vi "Begin[Conflict].vi"() -> (0 "Joystick 1 Error":errorcluster)   [LabVIEW 2013]
doc: "Called before other user functions, this VI is expected to open initial I/O refnums, load in file data, and do all program initialization. Notice that the <B>error out</B> terminal is simply used for data flow. Wiring it to other structures or subVIs ensures that this VI runs first."
uses:
  <vilib>/Rock Robotics/SystemInterfaces/DIO/FPGA_DIOPWMChannel.ctl
  <vilib>/Rock Robotics/WPI/SafetyOutput/WPI_SafetyOutputConfigMenu.ctl
  <vilib>/Rock Robotics/WPI/DriverStation/WPI_DriverStationRobotMode2.ctl
  <vilib>/Rock Robotics/SystemInterfaces/Typedef/FPGA_TypedefAnalogModuleForGyro.ctl
  <vilib>/Rock Robotics/SystemInterfaces/AI/FPGA_AIGyroChannel.ctl
  <vilib>/Rock Robotics/WPI/Solenoid/WPI_SolenoidChannel.ctl
  <vilib>/Rock Robotics/SystemInterfaces/DIO/FPGA_DIOChannel.ctl
  <vilib>/Rock Robotics/SystemInterfaces/DIO/FPGA_DIORelayChannel.ctl
  <vilib>/Rock Robotics/WPI/Relay/WPI_RelayDirection.ctl
  <vilib>/Rock Robotics/SystemInterfaces/Typedef/FPGA_TypedefSolenoidModule.ctl
  <vilib>/Rock Robotics/WPI/Joystick/WPI_JoystickDeviceEnum.ctl
  <vilib>/Rock Robotics/WPI/RobotDrive/WPI_RobotDriveOpen2MotorWithTalon.vi
  Robot Global Data.vi
  <vilib>/Rock Robotics/WPI/Solenoid/WPI_SolenoidOpenDouble.vi
panel:
  out "TestSolenoid56":errorcluster
  out "Test Gripper Error":errorcluster
  out "Right Solenoid Open Error":errorcluster
  out "Left Solenoid Open Error":errorcluster
  out "Extsionsion Solenoids Error":errorcluster
  out "Catapult Solenoids Error":errorcluster
  out "Gripper Solenoid Open Error":errorcluster
  out "Joystick 3 Error":errorcluster
  out "Gyro Open Error":errorcluster
  out "Joystick 1 Error 2":errorcluster
  out "Compressor Open Error":errorcluster
  out "Joystick 2 Error":errorcluster
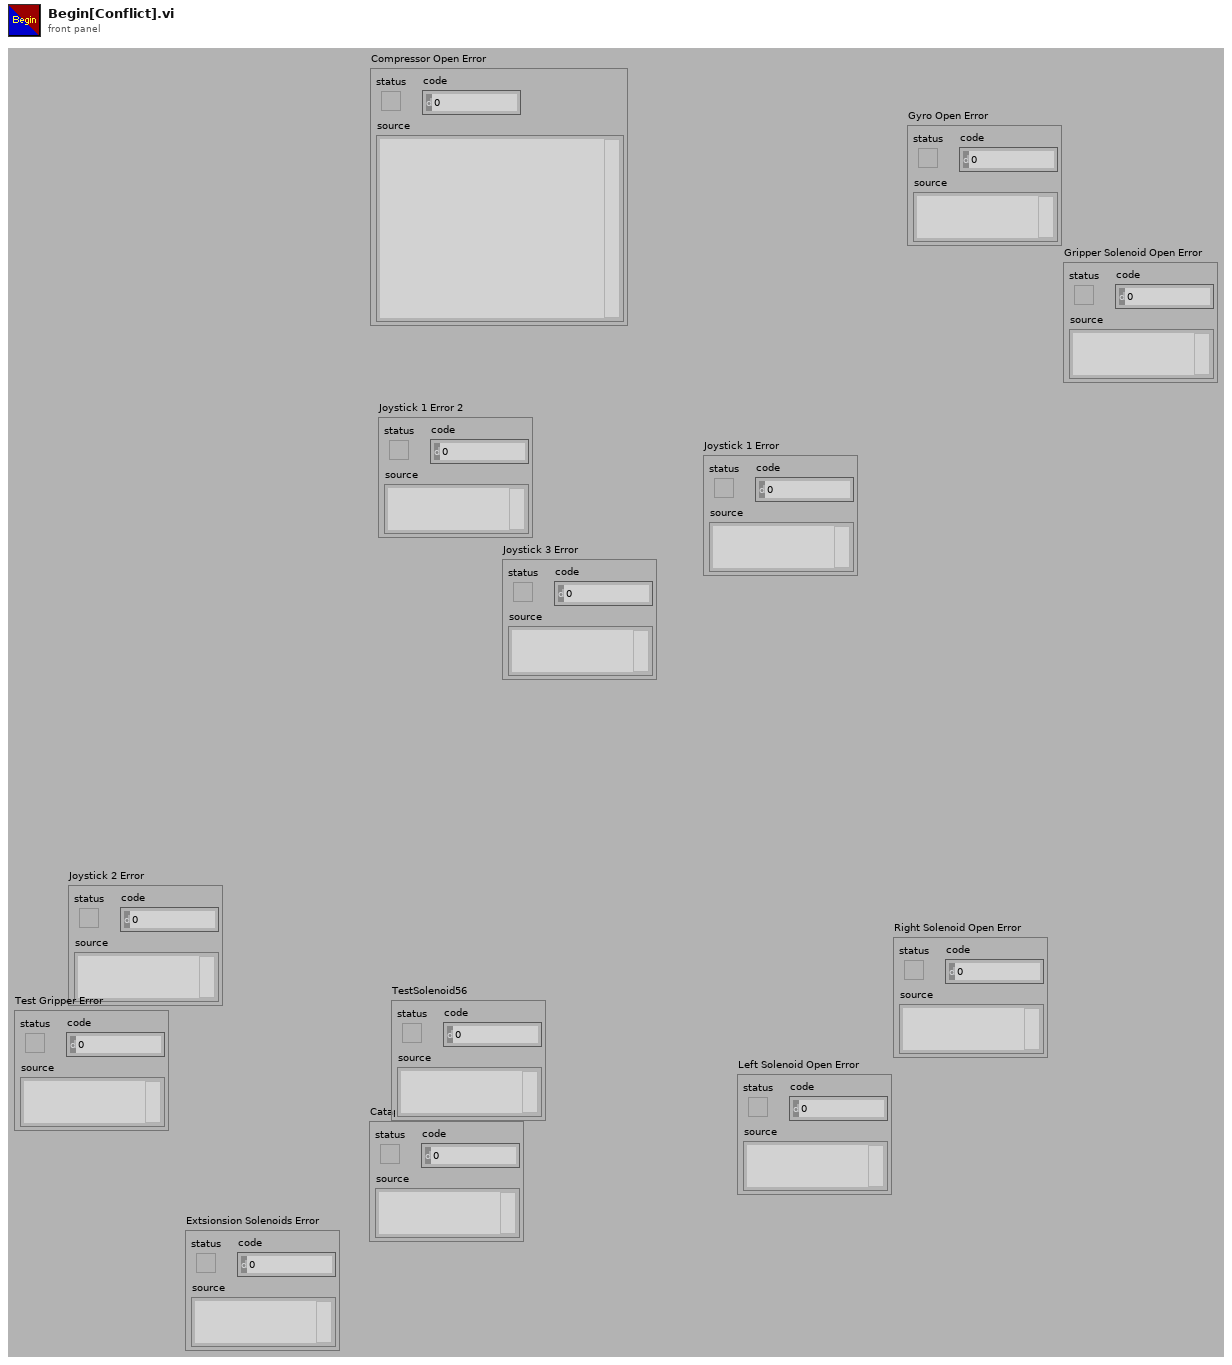
[diagram p1: front panel]
types:
  T1 = typedef "WPI_SolenoidChannel.ctl" = enum8{"Solenoid 1", "Solenoid 2", "Solenoid 3", "Solenoid 4", "Solenoid 5", "Solenoid 6", "Solenoid 7", "Solenoid 8", "Invalid"}
  T2 = typedef "FPGA_TypedefSolenoidModule.ctl" = enum16{"Solenoid Module 1", "Solenoid Module 2"}
  T3 = typedef "WPI_RelayDirection.ctl" = enum16{"Both directions", "Forward only", "Reverse only"}
  T4 = typedef "FPGA_DIORelayChannel.ctl" = enum8{"Relay 1", "Relay 2", "Relay 3", "Relay 4", "Relay 5", "Relay 6", "Relay 7", "Relay 8", "Invalid"}
  T5 = typedef "FPGA_DIOChannel.ctl" = enum8{"DIO 1", "DIO 2", "DIO 3", "DIO 4", "DIO 5", "DIO 6", "DIO 7", "DIO 8", "DIO 9", "DIO 10", "DIO 11", "DIO 12", "DIO 13", "DIO 14", "Invalid"}
  T6 = typedef "FPGA_AIGyroChannel.ctl" = enum8{"AI 1", "AI 2", "Invalid"}
  T7 = typedef "FPGA_TypedefAnalogModuleForGyro.ctl" = enum16{"Analog Module 1"}
  T8 = typedef "WPI_DriverStationRobotMode2.ctl" = enum16{"Autonomous Disabled", "Autonomous Enabled", "Teleop Disabled", "Teleop Enabled", "Timeout", "Finish", "Test Disabled", "Test Enabled"}
  T9 = typedef "WPI_SafetyOutputConfigMenu.ctl" = enum16{"Enable", "Disable"}
  T10 = typedef "FPGA_DIOPWMChannel.ctl" = enum8{"PWM 1", "PWM 2", "PWM 3", "PWM 4", "PWM 5", "PWM 6", "PWM 7", "PWM 8", "PWM 9", "PWM 10", "Invalid"}
  T11 = typedef "WPI_RobotDriveDevRef.ctl" = cluster{"DevStatus":errorcluster, "Motors[]":T12[], "Square Inputs":bool, "Max Output":dbl, "Isochronous":bool}
  T12 = typedef "WPI_MotorControlDeviceRef.ctl" = cluster{"DeviceStatus":errorcluster, "Type":enum16{"PWM", "CAN"}, "PWM":cluster{"Digital Module":T13, "PWM Channel":T10, "DeadBand":T14}, "CAN":cluster{"Device Number":u8, "Control Mode":T15, "Semaphore":T16, "Max Vout":dbl}, "Invert":bool, "TransformRef":T17, "InvTransformRef":T17}
  T13 = typedef "FPGA_TypedefDigitalModule.ctl" = enum16{"Digital Module 1", "Digital Module 2"}
  T14 = typedef "WPI_PWMDeadband.ctl" = cluster{"Name":string, "maxPositivePwm":i32, "minPositivePwm":i32, "centerPwm":i32, "maxNegativePwm":i32, "minNegativePwm":i32, "angularRange":u16}
  T15 = typedef "WPI_CANJaguar_ControlMode.ctl" = enum8{"Percent VBus", "Current", "Speed", "Position", "Voltage"}
  T16 = typedef "Semaphore RefNum" = refnum<k1>
  T17 = typedef "WPI_PWMTransform_ConPane.ctl" = refnum<vi>
  T18 = typedef "WPI_SolenoidDevRef.ctl" = cluster{"DevStatus":errorcluster, "Solenoid Module":T2, "Forward Solenoid Channel":T1, "Reverse Solenoid Channel":T1}
  T19 = typedef "WPI_JoystickDeviceEnum.ctl" = enum16{"USB 1", "USB 2", "USB 3", "USB 4", "Kinect 1", "Kinect 2"}
  T20 = typedef "WPI_JoystickDevRef.ctl" = cluster{"Device":T19}
  T21 = typedef "WPI_RelayDevRef.ctl" = cluster{"DevStatus":errorcluster, "Relay Channel":T4, "Digital Module":T13, "Relay Direction":T3}
  T22 = typedef "WPI_GyroDevRef.ctl" = cluster{"DevStatus":errorcluster, "Analog Module":T23, "Analog Channel":T24, "Offset":dbl, "Gain (VoltsPerDegree/Second)":dbl}
  T23 = typedef "FPGA_TypedefAnalogModule.ctl" = enum16{"Analog Module 1", "Analog Module 2"}
  T24 = typedef "FPGA_AIChannel.ctl" = enum8{"AI 1", "AI 2", "AI 3", "AI 4", "AI 5", "AI 6", "AI 7", "AI 8", "Invalid"}
  T25 = typedef "WPI_DigitalInputDevRef.ctl" = cluster{"DevStatus":errorcluster, "DIO Channel":T5, "Digital Module":T13}
  T26 = typedef "WPI_CompressorDevRef.ctl" = cluster{"DevStatus":errorcluster, "DigitalInputDevRef":T25, "RelayDevRef":T21}
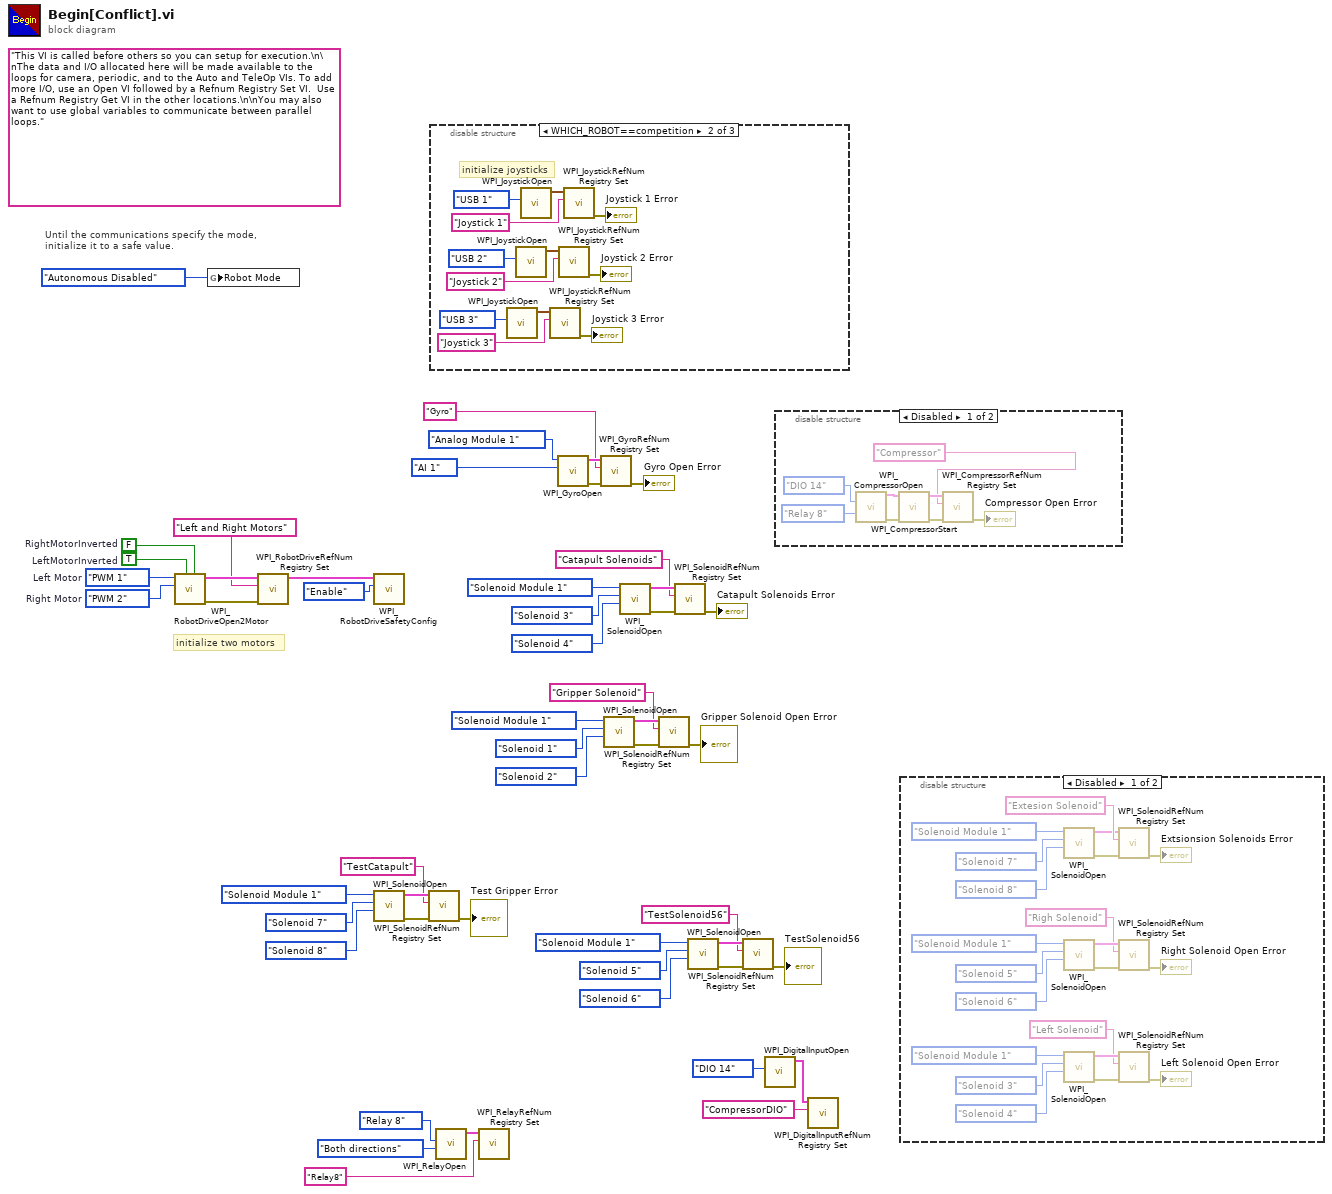
[diagram p0: block diagram]
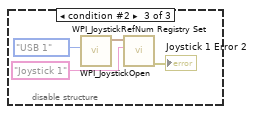
[diagram p5: hidden frame]
diagram:
  (unwired) "This VI is called before others so you can setup for execution.\n\nThe data and I/O allocated here will be made available to the loops for camera, periodic, and to the Auto and TeleOp VIs. To add more I/O, use an Open VI followed by a Refnum Registry Set VI.  Use a Refnum Registry Get VI in the other locations.\n\nYou may also want to use global variables to communicate between parallel loops."
  w45 = FPGA_DIOPWMChannel."PWM 2"  # Right Motor
  w46 = FPGA_DIOPWMChannel."PWM 1"  # Left Motor
  w50 = TRUE  # LeftMotorInverted
  w51 = FALSE  # RightMotorInverted
  # "Until the communications specify the mode,\ninitialize it to a safe value."
  # "initialize two motors"
  n1 = call-poly <vilib>:"WPI_RobotDriveOpen2Motor.vi"("Right Motor Inverted"=w51, "Left Motor Inverted"=w50, "Right Motor"=w45, "Left Motor"=w46) -> ("error out"=w47:errorcluster, "RobotDriveDevRef"=w49:T11)  [unwired: 1 in, 5 out]
  n2 = global write "Robot Global Data.vi" "Robot Mode"(WPI_DriverStationRobotMode2."Autonomous Disabled" ("Robot Mode")) -> ()
  n3 = call <vilib>:"WPI_RobotDriveRefNum Registry Set.vi"("error in (no error)"=w47, "refnum name"="Left and Right Motors", "RobotDriveDevRef"=w49) -> ("RobotDriveDevRef"=w44:T11)  [unwired: 8 out]
  n4 = call <vilib>:"WPI_RobotDriveSafetyConfig.vi"("mode"=WPI_SafetyOutputConfigMenu."Enable", "RobotDriveDevRef"=w44) -> ()  [unwired: 8 in, 2 out]
  n5 = call-poly <vilib>:"WPI_SolenoidOpen.vi"("Reverse Solenoid Channel"=WPI_SolenoidChannel."Solenoid 8", "Forward Solenoid Channel"=WPI_SolenoidChannel."Solenoid 7", "Solenoid Module (Module 1)"=FPGA_TypedefSolenoidModule."Solenoid Module 1") -> ("error out"=w10:errorcluster, "SolenoidDevRef"=w11:T18)  [unwired: 7 in]
  n6 = call <vilib>:"WPI_SolenoidRefNum Registry Set.vi"("error in (no error)"=w10, "refnum name"="TestCatapult", "SolenoidDevRef"=w11) -> ("error out"=→"Test Gripper Error":errorcluster)  [unwired: 7 in, 1 out]
  n7 = disable-structure shown="WHICH_ROBOT==competition" {
    frame condition #0 {
    }
    frame condition #1 (active) {
      # "initialize joysticks"
      n8 = call <vilib>:"WPI_JoystickOpen.vi"("JoystickDevice"=WPI_JoystickDeviceEnum."USB 3") -> ("JoystickDevRef"=w53:T20)  [unwired: 10 in]
      n9 = call <vilib>:"WPI_JoystickOpen.vi"("JoystickDevice"=WPI_JoystickDeviceEnum."USB 2") -> ("JoystickDevRef"=w61:T20)  [unwired: 10 in]
      n10 = call <vilib>:"WPI_JoystickOpen.vi"("JoystickDevice"=WPI_JoystickDeviceEnum."USB 1") -> ("JoystickDevRef"=w57:T20)  [unwired: 10 in]
      n11 = call <vilib>:"WPI_JoystickRefNum Registry Set.vi"("refnum name"="Joystick 3", "JoystickDevRef"=w53) -> ("error out"=→"Joystick 3 Error":errorcluster)  [unwired: 8 in, 1 out]
      n12 = call <vilib>:"WPI_JoystickRefNum Registry Set.vi"("refnum name"="Joystick 2", "JoystickDevRef"=w61) -> ("error out"=→"Joystick 2 Error":errorcluster)  [unwired: 8 in, 1 out]
      n13 = call <vilib>:"WPI_JoystickRefNum Registry Set.vi"("refnum name"="Joystick 1", "JoystickDevRef"=w57) -> ("error out"=→"Joystick 1 Error":errorcluster)  [unwired: 8 in, 1 out]
    }
    frame condition #2 {
      n14 = call <vilib>:"WPI_JoystickOpen.vi"("JoystickDevice"=WPI_JoystickDeviceEnum."USB 1") -> ("JoystickDevRef"=w65:T20)  [unwired: 10 in]
      n15 = call <vilib>:"WPI_JoystickRefNum Registry Set.vi"("refnum name"="Joystick 1", "JoystickDevRef"=w65) -> ("error out"=→"Joystick 1 Error 2":errorcluster)  [unwired: 8 in, 1 out]
    }
  }
  n16 = call <vilib>:"WPI_RelayOpen.vi"("Relay Direction"=WPI_RelayDirection."Both directions", "Relay Channel"=FPGA_DIORelayChannel."Relay 8") -> ("RelayDevRef"=w16:T21)  [unwired: 8 in, 1 out]
  n17 = call <vilib>:"WPI_RelayRefNum Registry Set.vi"("refnum name"="Relay8", "RelayDevRef"=w16) -> ()  [unwired: 8 in, 2 out]
  n18 = call <vilib>:"WPI_GyroOpen.vi"("Analog Channel"=FPGA_AIGyroChannel."AI 1", "Analog Module (Module 1)"=FPGA_TypedefAnalogModuleForGyro."Analog Module 1") -> ("error out"=w37:errorcluster, "GyroDevRef"=w39:T22)  [unwired: 7 in, 1 out]
  n19 = call <vilib>:"WPI_GyroRefNum Registry Set.vi"("error in (no error)"=w37, "refnum name"="Gyro", "GyroDevRef"=w39) -> ("error out"=→"Gyro Open Error":errorcluster)  [unwired: 7 in, 1 out]
  n20 = call-poly <vilib>:"WPI_SolenoidOpen.vi"("Reverse Solenoid Channel"=WPI_SolenoidChannel."Solenoid 2", "Forward Solenoid Channel"=WPI_SolenoidChannel."Solenoid 1", "Solenoid Module (Module 1)"=FPGA_TypedefSolenoidModule."Solenoid Module 1") -> ("error out"=w31:errorcluster, "SolenoidDevRef"=w32:T18)  [unwired: 7 in]
  n21 = call-poly <vilib>:"WPI_SolenoidOpen.vi"("Reverse Solenoid Channel"=WPI_SolenoidChannel."Solenoid 4", "Forward Solenoid Channel"=WPI_SolenoidChannel."Solenoid 3", "Solenoid Module (Module 1)"=FPGA_TypedefSolenoidModule."Solenoid Module 1") -> ("error out"=w25:errorcluster, "SolenoidDevRef"=w26:T18)  [unwired: 7 in]
  n22 = call <vilib>:"WPI_SolenoidRefNum Registry Set.vi"("error in (no error)"=w31, "refnum name"="Gripper Solenoid", "SolenoidDevRef"=w32) -> ("error out"=→"Gripper Solenoid Open Error":errorcluster)  [unwired: 7 in, 1 out]
  n23 = call <vilib>:"WPI_SolenoidRefNum Registry Set.vi"("error in (no error)"=w25, "refnum name"="Catapult Solenoids", "SolenoidDevRef"=w26) -> ("error out"=→"Catapult Solenoids Error":errorcluster)  [unwired: 7 in, 1 out]
  n24 = call-poly <vilib>:"WPI_SolenoidOpen.vi"("Reverse Solenoid Channel"=WPI_SolenoidChannel."Solenoid 6", "Forward Solenoid Channel"=WPI_SolenoidChannel."Solenoid 5", "Solenoid Module (Module 1)"=FPGA_TypedefSolenoidModule."Solenoid Module 1") -> ("error out"=w3:errorcluster, "SolenoidDevRef"=w4:T18)  [unwired: 7 in]
  n25 = call <vilib>:"WPI_SolenoidRefNum Registry Set.vi"("error in (no error)"=w3, "refnum name"="TestSolenoid56", "SolenoidDevRef"=w4) -> ("error out"=→"TestSolenoid56":errorcluster)  [unwired: 7 in, 1 out]
  n26 = call <vilib>:"WPI_DigitalInputOpen.vi"("DIO Channel"=FPGA_DIOChannel."DIO 14") -> ("DigitalInputDevRef"=w20:T25)  [unwired: 9 in, 1 out]
  n27 = disable-structure shown="Disabled" {
    frame Disabled {
      n28 = call <vilib>:"WPI_CompressorOpen.vi"("Pressure Switch DIO Channel"=FPGA_DIOChannel."DIO 14", "Relay Channel"=FPGA_DIORelayChannel."Relay 8") -> ("CompressorDevRef"=w73:T26, "error out"=w72:errorcluster)  [unwired: 12 in]
      n29 = call <vilib>:"WPI_CompressorStart.vi"("error in (no error)"=w72, "CompressorDevRef"=w73) -> ("error out"=w70:errorcluster, "CompressorDevRef"=w71:T26)  [unwired: 8 in]
      n30 = call <vilib>:"WPI_CompressorRefNum Registry Set.vi"("error in (no error)"=w70, "refnum name"="Compressor", "CompressorDevRef"=w71) -> ("error out"=→"Compressor Open Error":errorcluster)  [unwired: 7 in, 1 out]
    }
    frame Enabled {
    }
  }
  n31 = call <vilib>:"WPI_DigitalInputRefNum Registry Set.vi"("refnum name"="CompressorDIO", "DigitalInputDevRef"=w20) -> ()  [unwired: 8 in, 2 out]
  n32 = disable-structure shown="Disabled" {
    frame Disabled {
      n33 = call-poly <vilib>:"WPI_SolenoidOpen.vi"("Reverse Solenoid Channel"=WPI_SolenoidChannel."Solenoid 8", "Forward Solenoid Channel"=WPI_SolenoidChannel."Solenoid 7", "Solenoid Module (Module 1)"=FPGA_TypedefSolenoidModule."Solenoid Module 1") -> ("error out"=w79:errorcluster, "SolenoidDevRef"=w78:T18)  [unwired: 7 in]
      n34 = call-poly <vilib>:"WPI_SolenoidOpen.vi"("Reverse Solenoid Channel"=WPI_SolenoidChannel."Solenoid 6", "Forward Solenoid Channel"=WPI_SolenoidChannel."Solenoid 5", "Solenoid Module (Module 1)"=FPGA_TypedefSolenoidModule."Solenoid Module 1") -> ("error out"=w88:errorcluster, "SolenoidDevRef"=w89:T18)  [unwired: 7 in]
      n35 = call-poly <vilib>:"WPI_SolenoidOpen.vi"("Reverse Solenoid Channel"=WPI_SolenoidChannel."Solenoid 4", "Forward Solenoid Channel"=WPI_SolenoidChannel."Solenoid 3", "Solenoid Module (Module 1)"=FPGA_TypedefSolenoidModule."Solenoid Module 1") -> ("error out"=w93:errorcluster, "SolenoidDevRef"=w94:T18)  [unwired: 7 in]
      n36 = call <vilib>:"WPI_SolenoidRefNum Registry Set.vi"("error in (no error)"=w79, "refnum name"="Extesion Solenoid", "SolenoidDevRef"=w78) -> ("error out"=→"Extsionsion Solenoids Error":errorcluster)  [unwired: 7 in, 1 out]
      n37 = call <vilib>:"WPI_SolenoidRefNum Registry Set.vi"("error in (no error)"=w88, "refnum name"="Righ Solenoid", "SolenoidDevRef"=w89) -> ("error out"=→"Right Solenoid Open Error":errorcluster)  [unwired: 7 in, 1 out]
      n38 = call <vilib>:"WPI_SolenoidRefNum Registry Set.vi"("error in (no error)"=w93, "refnum name"="Left Solenoid", "SolenoidDevRef"=w94) -> ("error out"=→"Left Solenoid Open Error":errorcluster)  [unwired: 7 in, 1 out]
    }
    frame Enabled {
    }
  }
